vi "GetVersionSerializableData.vi"(10 "Version":u16, 11 "Bill Murray":refnum<class "Bill Murray.lvclass">) -> (0 "error out":errorcluster, 1 "Found?":bool, 2 "SerializableData":variant, 3 "Bill Murray":refnum<class "Bill Murray.lvclass">)   [LabVIEW 2020, in "Bill Murray.lvclass"]
uses:
  Bill Murray.lvclass
  SerializableData_v1.ctl
  Golf Club.lvclass
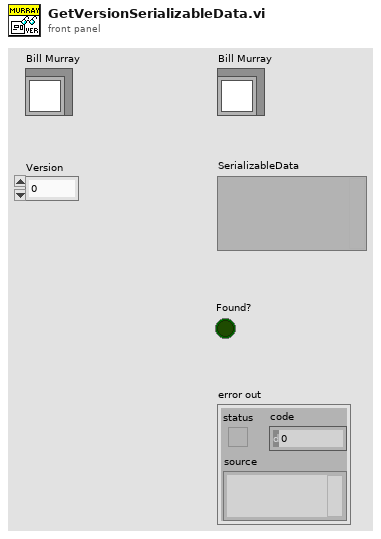
[diagram p1: front panel]
types:
  T1 = typedef "Bill Murray.lvclass/SerializableData_v1.ctl" = cluster{"Nickname":string, "Golf Club":refnum<class "Golf Club.lvclass">}
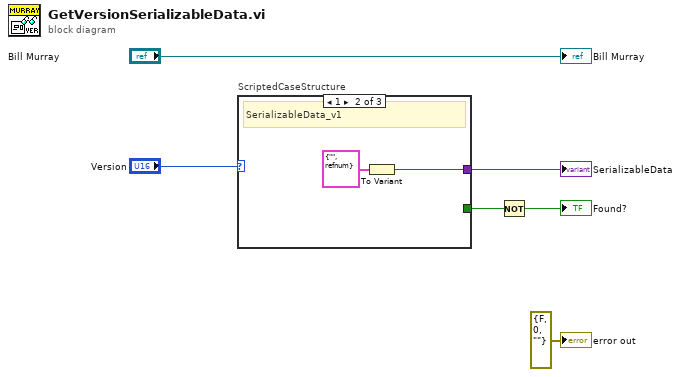
[diagram p0: block diagram]
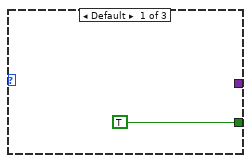
[diagram p2: hidden frame]
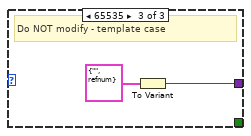
[diagram p3: hidden frame]
diagram:
  n1 = case "ScriptedCaseStructure" shown="1" "Version" {
    tunnel: [_ w9 w11] -> w5
    tunnel: [TRUE _ _] -> w4
    frame Default {
    }
    frame 1 {
      # "SerializableData_v1"
      n2 = To Variant(anything=T1 {"Nickname"="", "Golf Club"=refnum} ("SerializableData")) -> (Variant=w9:variant)
    }
    frame 65535 {
      # "Do NOT modify - template case"
      n3 = To Variant(anything=T1 {"Nickname"="", "Golf Club"=refnum} ("SerializableData")) -> (Variant=w11:variant)
    }
  }
  "SerializableData" <- w5
  n4 = Not(x=w4) -> (.not. x?=→"Found?":bool)
  "error out" <- errorcluster {"status"=FALSE, "code"=0, "source"=""} ("error out")
  "Bill Murray" <- "Bill Murray"
